vi "Init_Instr.vi"(8 "error in (no error)":errorcluster caption="entrée d'erreur (pas d'erreur)", 11 "Class DIO en entrée":refnum<class "Class Instrument Ana.lvclass">) -> (0 "error out":errorcluster caption="sortie d'erreur", 3 "Class DIO en Sortie":refnum<class "Class Instrument Ana.lvclass">)   [LabVIEW 2020, in "Library Instrument & Equipement.lvlib" / "Library Instruments.lvlib" / "Class Instrument Ana.lvclass"]
uses:
  Class Instrument Ana.lvclass
  Class Instrument Ana.lvclass/Class Instrument Ana.ctl
  Instrument (Default)/Class Instrument (Default).lvclass
  Ana/Class Ana (Default)/Class Ana (Default).lvclass
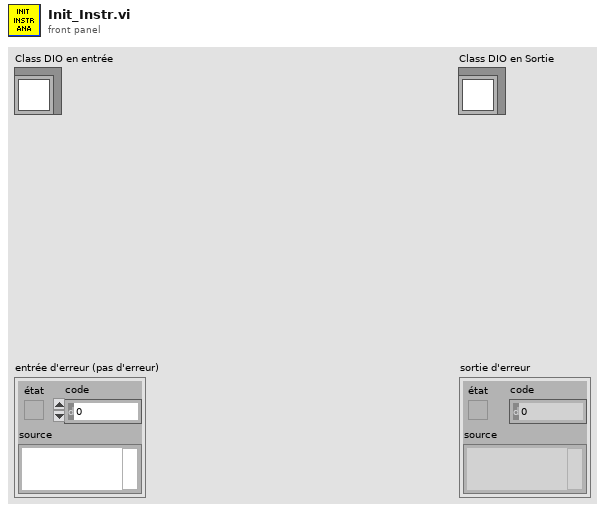
[diagram p1: front panel]
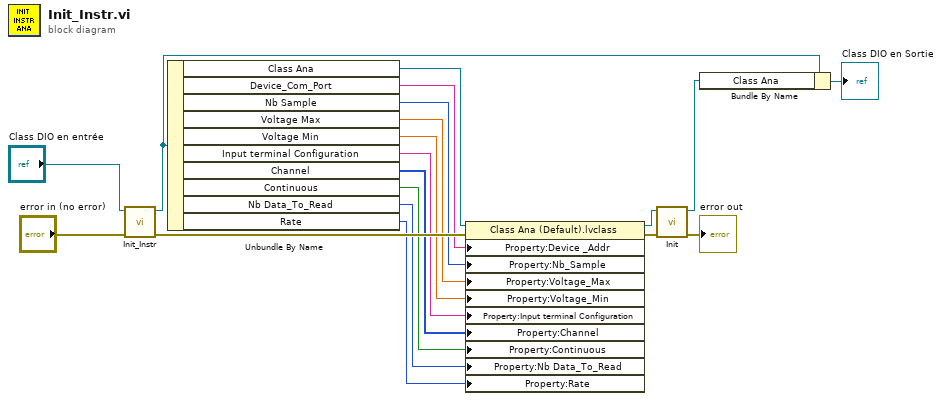
[diagram p0: block diagram]
diagram:
  n1 = call-parent "Init_Instr.vi"("error in (no error)"="error in (no error)", "Class Instrument (Default) en entrée"="Class DIO en entrée") -> ("error out"=w13:errorcluster, "Class Instrument (Default) en sortie"=w14:refnum<class "Class Instrument Ana.lvclass">)  [unwired: 8 in]
  n2 = Unbundle By Name(w14) -> ("Class Ana"=w12:refnum<class "Class Ana (Default).lvclass">, "Device_Com_Port"=w9:string, "Nb Sample"=w8:u16, "Voltage Max"=w7:dbl, "Voltage Min"=w6:dbl, "Input terminal Configuration"=w5:string, "Channel"=w4:u8[], "Continuous"=w3:bool, "Nb Data_To_Read"=w2:i16, "Rate"=w1:u16)
  n3 = property class="Class Ana (Default).lvclass"(reference=w12, error in=w13, "Property:Device _Addr"=w9, "Property:Nb_Sample"=w8, "Property:Voltage_Max"=w7, "Property:Voltage_Min"=w6, "Property:Input terminal Configuration"=w5, "Property:Channel"=w4, "Property:Continuous"=w3, "Property:Nb Data_To_Read"=w2, "Property:Rate"=w1) -> (reference out=w11:refnum<class "Class Ana (Default).lvclass">, error out=w10:errorcluster)
  n4 = call-dynamic "Init.vi"("error in (no error)"=w10, "Class DIO (Default) en entrée"=w11) -> ("error out"=→"error out":errorcluster, "Class DIO (Default) en sortie"=w15:refnum<class "Class Ana (Default).lvclass">)  [unwired: 8 in]
  n5 = Bundle By Name(cluster=w14, "Class Ana"=w15) -> (→"Class DIO en Sortie":refnum<class "Class Instrument Ana.lvclass">)
